vi "generate table.vi"(5 "assemblies":refnum<vi>, 7 "table":refnum<vi>, 8 "error in":errorcluster, 10 "engine configuration in":refnum<class "engine configuration.lvclass">, 11 "EthernetIP configuration in":refnum<class "EthernetIP configuration.lvclass">) -> (0 "error out":errorcluster)   [LabVIEW 2013, in "EthernetIP editor node.lvclass"]
uses:
  EthernetIP editor node.lvclass
  <vilib>/NI/TBM Modules/Ethernet IP/configuration/EthernetIP configuration.lvclass
  <vilib>/NI/Module Execution Interface/Engine Configuration/engine configuration.lvclass
  <vilib>/NI/Tag Bus Module Framework/root configuration/TBM configuration.lvclass/TBM configuration.ctl
  <vilib>/NI/TBM Modules/Ethernet IP/configuration/EthernetIP configuration.lvclass/EthernetIP configuration.ctl
  table line.ctl
  <vilib>/NI/TBM Modules/Ethernet IP/channel/EthernetIP Channel.lvclass
  <vilib>/NI/Tag Bus/tag/tag descriptor.lvclass/tag descriptor.ctl
  <vilib>/NI/Tag Bus/tag/read tag name.vi
  <vilib>/NI/Tag Bus Module Framework/root configuration/Read instance name.vi
  <vilib>/NI/TBM Modules/Ethernet IP/configuration/read eip channels.vi
  <vilib>/NI/TBM Modules/Ethernet IP/configuration/Read assemblies.vi
  <vilib>/NI/Tag Bus Module Framework/root configuration/create GUID.vi
  <vilib>/NI/Tag Bus/tag/tag descriptor.lvclass
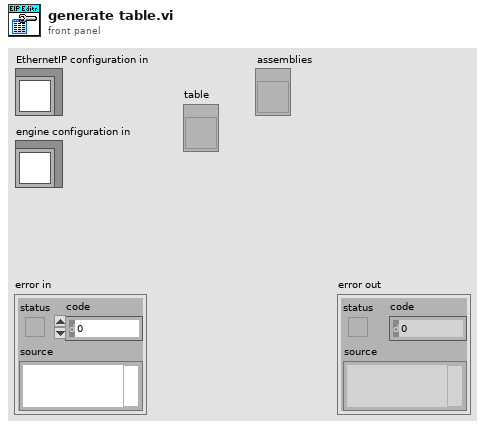
[diagram p1: front panel]
types:
  T1 = typedef "EthernetIP configuration.lvclass/assembly definition.ctl" = cluster{"name":string, "Instance ID":u32, "Type":T2, "Size (bytes)":u32, "big endian?":bool}
  T2 = typedef "EthernetIP configuration.lvclass/assembly type.ctl" = enum32{"Producing", "Consuming"}
  T3 = typedef "EthernetIP editor node.lvclass/table line.ctl" = cluster{"eip channels":refnum<class "EthernetIP Channel.lvclass">, "tag name":string}
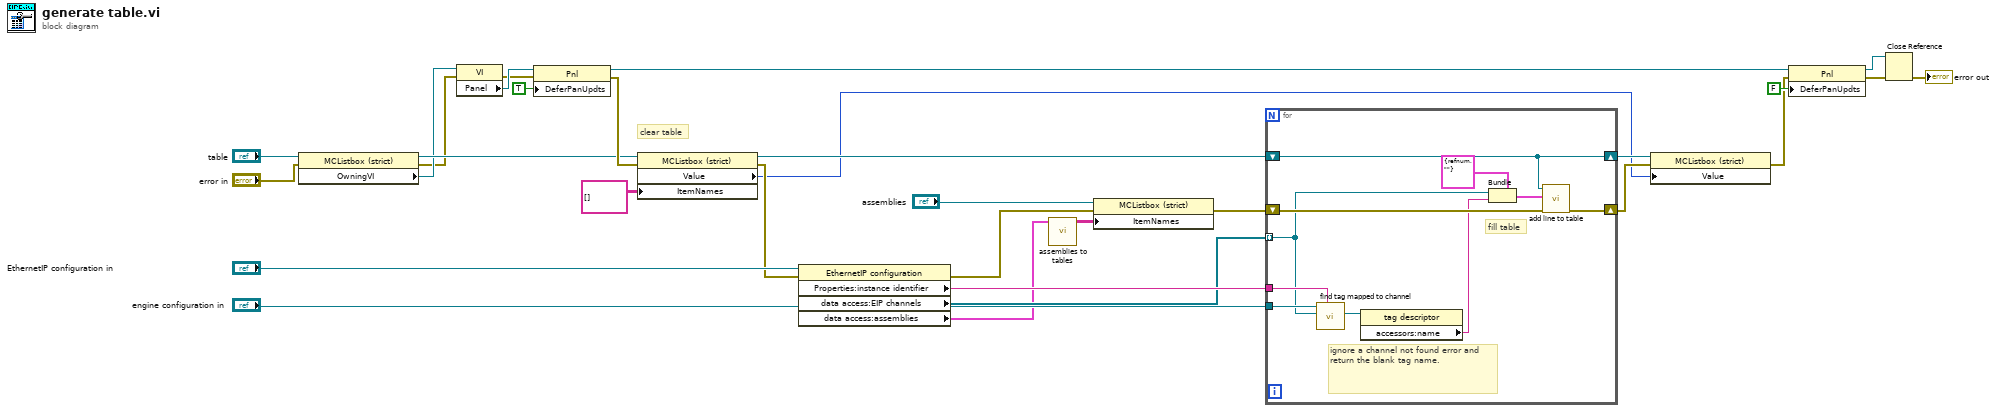
[diagram p0: block diagram]
diagram:
  # "clear table"
  n1 = property class="MCListbox (strict)"(reference="table", error in="error in") -> (reference out=w12:refnum<vi>, error out=w9:errorcluster, "OwningVI"=w10:refnum<vi>)
  n2 = property class="VI"(reference=w10, error in=w9) -> (error out=w18:errorcluster, "Panel"=w19:refnum<vi>)  [unwired: 1 out]
  n3 = property class="Pnl"(reference=w19, error in=w18, "DeferPanUpdts"=TRUE ("Defer Panel Updates")) -> (reference out=w15:refnum<vi>, error out=w17:errorcluster)
  n4 = property class="MCListbox (strict)"(reference=w12, error in=w17, "ItemNames"=string[][] [] ("Item Names")) -> (reference out=w29:refnum<vi>, error out=w25:errorcluster, "Value"=w21:i32)
  n5 = property class="EthernetIP configuration"(reference="EthernetIP configuration in", error in=w25) -> (error out=w4:errorcluster, "Properties:instance identifier"=w26:string, "data access:EIP channels"=w6:refnum<class "EthernetIP Channel.lvclass">[], "data access:assemblies"=w5:T1[])  [unwired: 1 out]
  n6 = call "assemblies to tables.vi"("assemblies"=w5) -> ("Item Names"=w1:string[][])  [unwired: 10 in]
  n7 = property class="MCListbox (strict)"(reference="assemblies", error in=w4, "ItemNames"=w1) -> (error out=w3:errorcluster)  [unwired: 1 out]
  n8 = for {
    shift-right: [w40] -> w22
    shift-left: w3 -> [w37]
    tunnel: w6 -> [w34] mode=indexing
    tunnel: "engine configuration in" -> [w36]
    tunnel: w26 -> [w35]
    shift-right: [w31] -> w23
    shift-left: w29 -> [w31]
    # "ignore a channel not found error and return the blank tag name."
    # "fill table"
    n9 = call <vilib>:"find tag mapped to channel.vi"("owner"=w35, "channel"=w34, "engine configuration in"=w36) -> ("tag"=w33:refnum<class "tag descriptor.lvclass">)  [unwired: 6 in, 2 out]
    n10 = property class="tag descriptor"(reference=w33) -> ("accessors:name"=w32:string)  [unwired: 1 in, 2 out]
    n11 = Bundle(cluster=T3 {"eip channels"=refnum, "tag name"=""} ("line"), "eip channels"=w34, "tag name"=w32) -> (w38:T3)
    n12 = call "add line to table.vi"("error in"=w37, "line"=w38, "operations table"=w31) -> ("error out"=w40:errorcluster)  [unwired: 8 in]
  }
  n13 = property class="MCListbox (strict)"(reference=w23, error in=w22, "Value"=w21) -> (error out=w14:errorcluster)  [unwired: 1 out]
  n14 = property class="Pnl"(reference=w15, error in=w14, "DeferPanUpdts"=FALSE ("Defer Panel Updates")) -> (reference out=w7:refnum<vi>, error out=w13:errorcluster)
  n15 = Close Reference(reference=w7, error in (no error)=w13) -> (error out=→"error out":errorcluster)
